vi "BoxShootPID.vi"(6 "Auto":bool=TRUE, 9 "FPGA_Time_Seconds":dbl=-1.0, 10 "Setpoint":dbl, 11 "Sensor Velocity":dbl) -> (0 "Filtered Velocity":dbl format="%13.5p", 1 "FeedForward":dbl, 2 "AtSetpoint":bool, 3 "CO-ControlOutput":dbl)   [LabVIEW 2023]
uses:
  <vilib>/Rock Robotics/WPI/ThirdParty/JAS_Junk/TrajLib/LinearFilter_ResetToValue.vi
  <vilib>/Rock Robotics/WPI/ThirdParty/JAS_Junk/TrajLib/LinearFilter_Calculate.vi
  <vilib>/Rock Robotics/WPI/ThirdParty/JAS_Junk/TrajLib/SimpleMotorFF_Calculate.vi
  <vilib>/Rock Robotics/WPI/ThirdParty/JAS_Junk/TrajLib/PIDController_AtSetpoint.vi
  <vilib>/Rock Robotics/WPI/ThirdParty/JAS_Junk/TrajLib/PIDController_SetPIDF.vi
  <vilib>/Rock Robotics/WPI/ThirdParty/JAS_Junk/TrajLib/PIDController_SetDerivativeFilter.vi
  <vilib>/Rock Robotics/WPI/ThirdParty/JAS_Junk/TrajLib/PIDController_SetIntegratorRange.vi
  <vilib>/Rock Robotics/WPI/ThirdParty/JAS_Junk/TrajLib/PIDController_SetTolerancePandV.vi
  <vilib>/Rock Robotics/WPI/ThirdParty/JAS_Junk/TrajLib/PIDController_DisableContinousInput.vi
  <vilib>/Rock Robotics/WPI/ThirdParty/JAS_Junk/TrajLib/PIDController_EnableContinousInput.vi
  <vilib>/Rock Robotics/WPI/ThirdParty/JAS_Junk/TrajLib/PIDController_Reset.vi
  <vilib>/Rock Robotics/WPI/ThirdParty/JAS_Junk/TrajLib/PIDController_New.vi
  <vilib>/Rock Robotics/WPI/ThirdParty/JAS_Junk/TrajLib/PIDController_SetOutputLimits.vi
  <vilib>/Rock Robotics/WPI/ThirdParty/JAS_Junk/TrajLib/PIDController_NewPeriod.vi
  <vilib>/Rock Robotics/SystemInterfaces/NetworkCommunication/NetComm_UsageReport_report.vi
  <vilib>/Rock Robotics/WPI/ThirdParty/JAS_Junk/TrajLib/LinearFilter_MovingAverage.vi
  <vilib>/Rock Robotics/WPI/ThirdParty/JAS_Junk/TrajLib/LinearFilter_LowPassBW1.vi
  <vilib>/Rock Robotics/WPI/ThirdParty/JAS_Junk/TrajLib/LinearFilter_LowPassBW2.vi
  <vilib>/Rock Robotics/WPI/ThirdParty/JAS_Junk/TrajLib/LinearFilter_HighPassBW1.vi
  <vilib>/Rock Robotics/WPI/ThirdParty/JAS_Junk/TrajLib/LinearFilter_HighPassBW2.vi
  <vilib>/Rock Robotics/WPI/ThirdParty/JAS_Junk/TrajLib/Globals/Util_LibraryGlobals.vi
  <vilib>/Rock Robotics/WPI/ThirdParty/JAS_Junk/TrajLib/PIDController_AdvCalculate_FF_Sp_Pv.vi
  <vilib>/Rock Robotics/WPI/ThirdParty/JAS_Junk/TrajLib/Trajectory_Library.lvlib
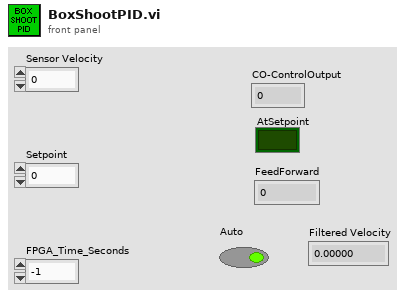
[diagram p1: front panel]
types:
  T1 = enum16{"Moving Average", "Low Pass 1st Order Butterworth", "Low Pass 2nd Order Butterworth", "High Pass 1st Order Butterworth", "High Pass 2nd Order Butterworth"}
  T2 = typedef "Trajectory_Library.lvlib/SIMPLE_MOTOR_FF.ctl" = cluster{"Ks":dbl, "Kv":dbl, "Ka":dbl, "KnInv":dbl}
  T3 = typedef "Trajectory_Library.lvlib/PID_ERROR_TOLERANCE.ctl" = cluster{"PositionTolerance":dbl, "VelocityTolerance":dbl}
  T4 = typedef "Trajectory_Library.lvlib/PID_ADV_LIMITS.ctl" = cluster{"MaxInput":dbl, "MinInput":dbl, "Continuous":bool, "MaxOutput":dbl, "MinOutput":dbl}
  T5 = typedef "Trajectory_Library.lvlib/PID_ADV_TUNING.ctl" = cluster{"Kf":dbl, "Kp":dbl, "Ki":dbl, "Kd":dbl, "MaximumIntegral":dbl, "MinimumIntegral":dbl, "Filter Derivative":bool}
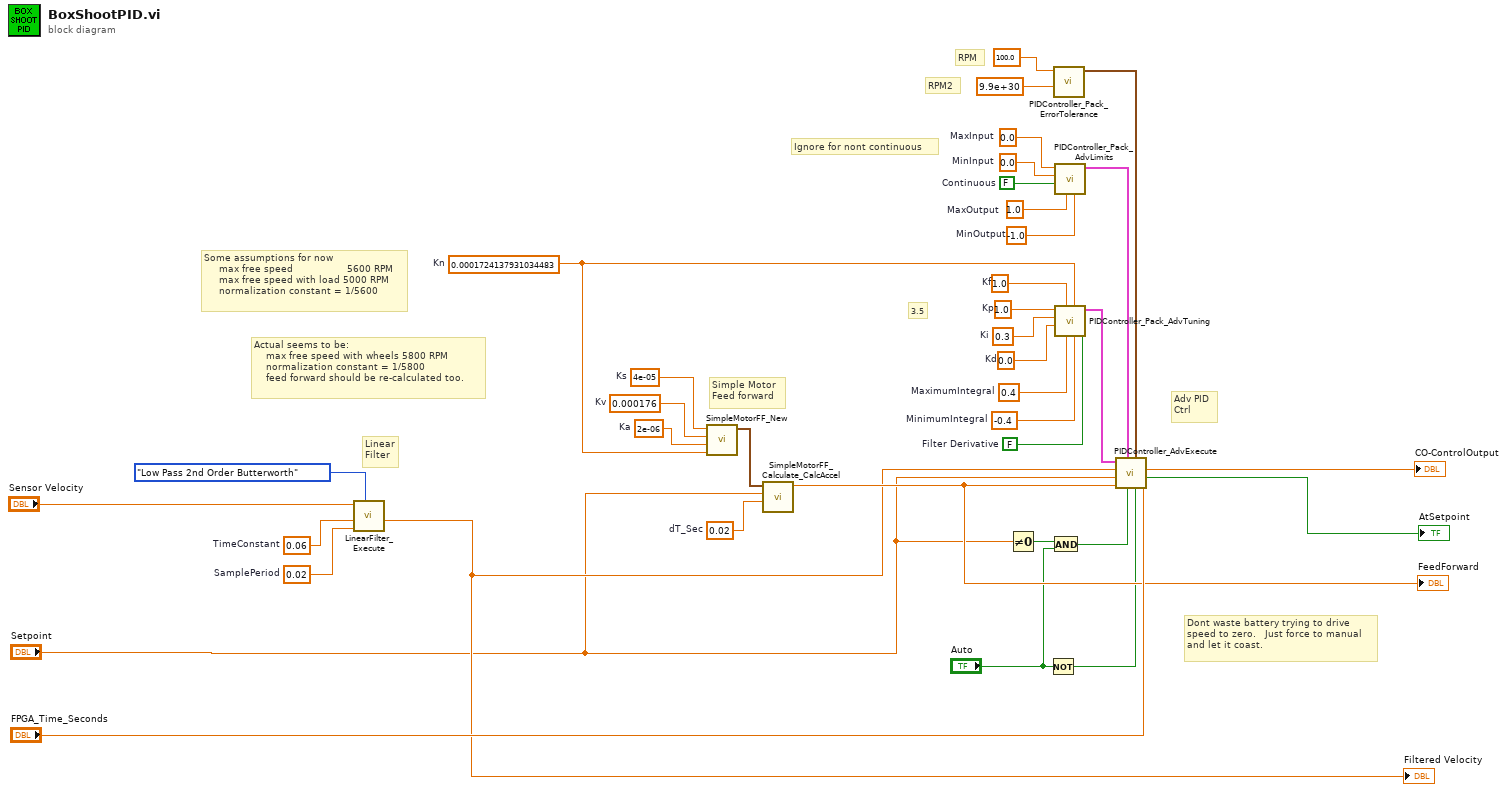
[diagram p0: block diagram]
diagram:
  w10 = 0.02  # SamplePeriod
  w9 = 0.06  # TimeConstant
  w17 = 1.0  # Kp
  w18 = 0.3  # Ki
  w19 = 0.0  # Kd
  w20 = 1.0  # Kf
  w21 = 0.4  # MaximumIntegral
  w22 = -0.4  # MinimumIntegral
  w23 = FALSE  # Filter Derivative
  w25 = 0.0  # MinInput
  w26 = FALSE  # Continuous
  w27 = 1.0  # MaxOutput
  w24 = -1.0  # MinOutput
  w28 = 0.0  # MaxInput
  w31 = 0.0001724137931034483  # Kn
  w12 = 0.02  # dT_Sec
  w14 = 4e-05  # Ks
  w15 = 0.000176  # Kv
  w16 = 2e-06  # Ka
  # "3.5"
  # "Dont waste battery trying to drive\nspeed to zero.   Just force to manual\nand let it coast."
  # "Actual seems to be:\n    max free speed with wheels 5800 RPM\n    normalization constant = 1/5800\n    feed forward should be re-calculated too."
  # "Linear\nFilter"
  # "RPM2"
  # "RPM"
  # "Some assumptions for now\n     max free speed                  5600 RPM\n     max free speed with load 5000 RPM\n     normalization constant = 1/5600"
  # "Ignore for nont continuous"
  # "Adv PID\nCtrl"
  # "Simple Motor\nFeed forward"
  n1 = call <vilib>:"LinearFilter_Execute.vi"("Filter Type"=T1."Low Pass 2nd Order Butterworth", "SamplePeriod"=w10, "TimeConstant"=w9, "Input"="Sensor Velocity") -> ("Output"=w6:dbl)  [unwired: 6 in, 1 out]
  "Filtered Velocity" <- w6
  n2 = call <vilib>:"SimpleMotorFF_New.vi"("Kn"=w31, "Ka"=w16, "Kv"=w15, "Ks"=w14) -> ("SIMPLE_MOTOR_FF"=w13:T2)  [unwired: 7 in]
  n3 = call <vilib>:"SimpleMotorFF_Calculate_CalcAccel.vi"("dT_Sec"=w12, "VelSp"="Setpoint", "SIMPLE_MOTOR_FF"=w13) -> ("FeedForward"=w32:dbl)  [unwired: 8 in]
  "FeedForward" <- w32
  n4 = Not Equal To 0?(x="Setpoint") -> (x != 0?=w5:bool)
  n5 = Not(x="Auto") -> (.not. x?=w1:bool)
  n6 = And(x=w5, y="Auto") -> (x .and. y?=w4:bool)
  n7 = call <vilib>:"PIDController_Pack_ErrorTolerance.vi"("VelocityTolerance"=9.9e+30, "PositionTolerance"=100.0) -> ("PID Error Tolerance"=w33:T3)  [unwired: 9 in]
  n8 = call <vilib>:"PIDController_Pack_AdvLimits.vi"("MinOutput"=w24, "MaxOutput"=w27, "Continuous"=w26, "MinInput"=w25, "MaxInput"=w28) -> ("Adv PID Limits"=w30:T4)  [unwired: 6 in]
  n9 = call <vilib>:"PIDController_Pack_AdvTuning.vi"("Filter Derivative"=w23, "MinimumIntegral"=w22, "Kn"=w31, "MaximumIntegral"=w21, "Kf"=w20, "Kd"=w19, "Ki"=w18, "Kp"=w17) -> ("Adv PID Tuning"=w29:T5)  [unwired: 3 in]
  n10 = call <vilib>:"PIDController_AdvExecute.vi"("Time"="FPGA_Time_Seconds", "Reset"=w1, "PID Error Tolerance"=w33, "Auto"=w4, "Adv PID Limits"=w30, "FF-FeedForward"=w32, "SP-SetPoint"="Setpoint", "PV-Measurement"=w6, "Adv PID Tuning"=w29) -> ("AtSetpoint"=→"AtSetpoint":bool, "CO-ControlOutput"=→"CO-ControlOutput":dbl)  [unwired: 1 out]
